vi "XCite_Only_Example.vi"() -> ()   [LabVIEW 2019]
doc: "This example demonstrates basic control of an X-Cite® light source. The first four channels of a connected light source can be switched on or off, and the power level adjusted. Note that this example will not be fail save, i.e. doesnt react on errors, just handles them forward to the end\n\nUsage:\n\nA search for X-Cite® devices is started, and if found controls are initialized for each channel. Channels can be switched on and off, and the intensity adjusted. To end the program click on \"quit\". All X-Cite® channels are switched off on exit."
uses:
  xcite/Xcite.lvclass
panel:
  out "error_out":errorcluster {"code" format="%.0x"}
  in  "quit":bool
  out "number_of_channels":i32
  in  "Power4":dbl
  out "Wavelength4":u32
  in  "Channel4":bool caption="wavelength"
  in  "Power3":dbl
  out "Wavelength3":u32
  in  "Channel3":bool caption="wavelength"
  in  "Power2":dbl
  out "Wavelength2":u32
  in  "Channel2":bool caption="wavelength"
  in  "Power1":dbl
  out "Wavelength1":u32
  in  "Channel1":bool caption="wavelength"
  out "display_name":string
  # "This example demonstrates basic control of an X-Cite® light source. The first four channels of a connected light source can be switched on or off, and the power level adjusted. Note that this example will not be fail save, i.e. doesnt react on errors, just handles them forward to the end\n\nUsage:\n\nA search for X-Cite® devices is started, and if found controls are initialized for each channel. Channels can be switched on and off, and the intensity adjusted. To end the program click on \"quit\". All X-Cite® channels are switched off on exit."
  # "pco.labview"
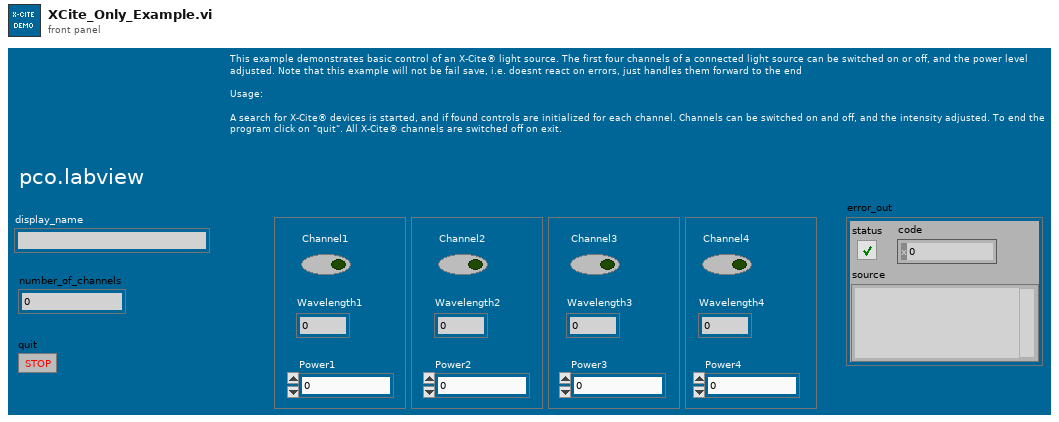
[diagram p1: front panel]
types:
  T1 = cluster{"serial":u32, "type":u16, "name":string, "wavelenghts_vec":u32[], "exclusivity_vec":u32[], "intensity_max_vec":u32[], "intensity_min_vec":u32[]}
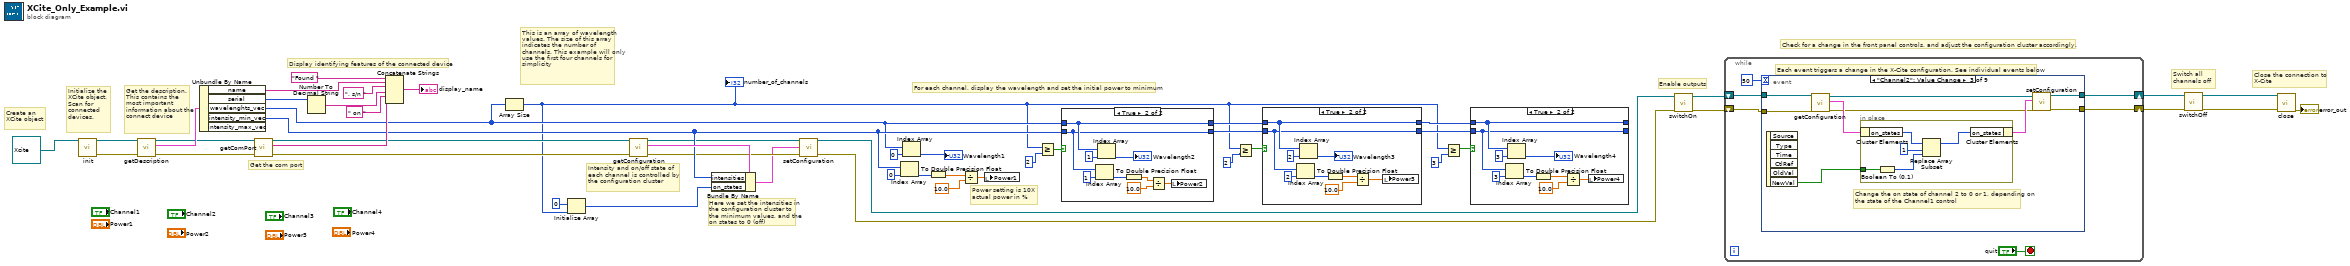
[diagram p0: block diagram]
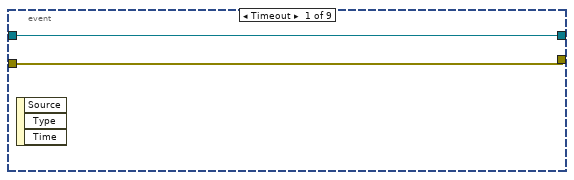
[diagram p2: hidden frame]
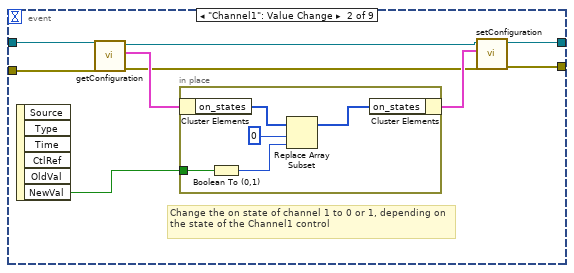
[diagram p3: hidden frame]
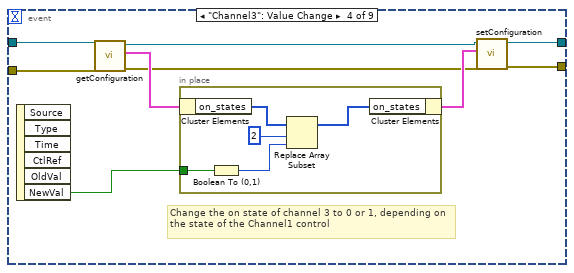
[diagram p4: hidden frame]
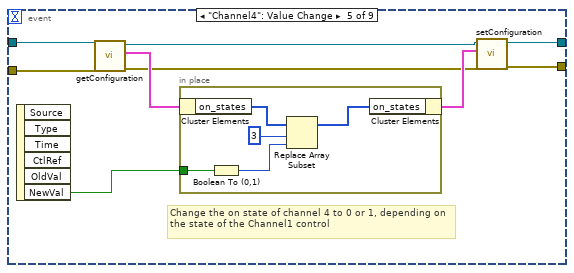
[diagram p5: hidden frame]
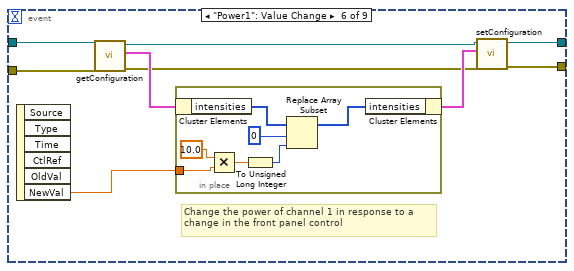
[diagram p6: hidden frame]
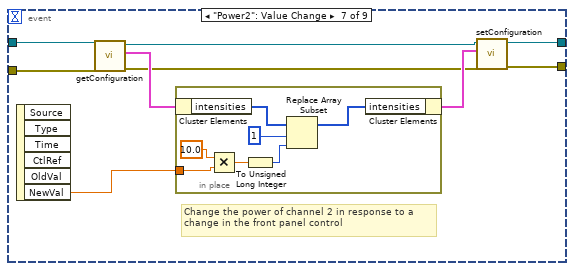
[diagram p7: hidden frame]
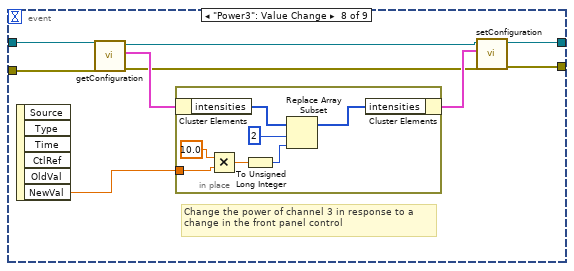
[diagram p8: hidden frame]
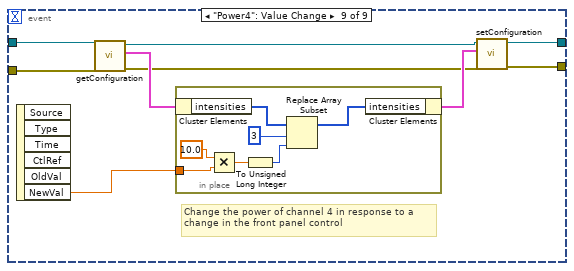
[diagram p9: hidden frame]
diagram:
  # "Enable outputs"
  # "Close the connection to X-Cite"
  # "Switch all channels off"
  # "Check for a change in the front panel controls, and adjust the configuration cluster accordingly."
  # "Power setting is 10X actual power in %"
  # "Here we set the intensities in the configuration cluster to the minimum values, and the on states to 0 (off)"
  # "Intensity and on/off state of each channel is controlled by the configuration cluster"
  # "For each channel, display the wavelength and set the initial power to minimum"
  # "This is an array of wavelength values. The size of this array indicates the number of channels. This example will only use the first four channels for simplicity"
  # "Display identifying features of the connected device"
  # "Get the com port"
  # "Get the description. This contains the most important information about the connect device"
  # "Initialize the XCite object. Scan for connected devices."
  # "Create an XCite object"
  n1 = call "init.vi"("Xcite in"=refnum<class "Xcite.lvclass"> refnum ("Xcite.lvclass")) -> ("error out"=w49:errorcluster, "Xcite out"=w50:refnum<class "Xcite.lvclass">)  [unwired: 9 in]
  n2 = call "getDescription.vi"("error in (no error)"=w49, "Xcite in"=w50) -> ("error out"=w45:errorcluster, "description"=w48:T1, "Xcite out"=w44:refnum<class "Xcite.lvclass">)  [unwired: 7 in]
  n3 = Unbundle By Name(w48) -> ("name"=w47:string, "serial"=w42:u32, "wavelenghts_vec"=w15:u32[], "intensity_min_vec"=w19:u32[])  [unwired: 1 out]
  n4 = call "getComPort.vi"("error in (no error)"=w45, "Xcite in"=w44) -> ("error out"=w21:errorcluster, "com_port"=w39:string, "Xcite out"=w22:refnum<class "Xcite.lvclass">)  [unwired: 7 in]
  n5 = Number To Decimal String(number=w42) -> (decimal integer string=w41:string)  [unwired: 1 in]
  n6 = Concatenate Strings("Found ", w47, ", s/n " ("string"), w41, " on " ("string"), w39) -> (→"display_name":string)
  n7 = Array Size(array=w15) -> (size(s)=w13:i32)
  "number_of_channels" <- w13
  n8 = Initialize Array(u8 0, w13) -> (w12:u8[])
  n9 = call "getConfiguration.vi"("error in (no error)"=w21, "Xcite in"=w22) -> ("error out"=w17:errorcluster, "configuration"=w20:cluster{"intensities":u32[], "on_states":u8[]}, "Xcite out"=w18:refnum<class "Xcite.lvclass">)  [unwired: 7 in]
  n10 = Bundle By Name(cluster=w20, "intensities"=w19, "on_states"=w12) -> (w16:cluster{"intensities":u32[], "on_states":u8[]})
  n11 = call "setConfiguration.vi"("error in (no error)"=w17, "configuration"=w16, "Xcite in"=w18) -> ("error out"=w2:errorcluster, "Xcite out"=w4:refnum<class "Xcite.lvclass">)  [unwired: 7 in]
  n12 = Index Array(array=w19, index=0) -> (element=w34:u32)
  n13 = Index Array(array=w15, index=0) -> (element=→"Wavelength1":u32)
  n14 = To Double Precision Float(number=w34) -> (double precision float=w33:dbl)
  n15 = Divide(x=w33, y=10.0) -> (x/y=w11:dbl)
  n16 = local write "Power1"(w11) -> ()
  n17 = Greater Or Equal?(x=w13, y=2) -> (x >= y?=w31:bool)
  n18 = case shown="True" w31 {
    tunnel: w15 -> [w53 w58]
    tunnel: w19 -> [w52 w57]
    tunnel: [w53 w58] -> w30
    tunnel: [w52 w57] -> w29
    frame False {
    }
    frame True {
      n19 = Index Array(array=w57, index=1) -> (element=w62:u32)
      n20 = Index Array(array=w58, index=1) -> (element=→"Wavelength2":u32)
      n21 = To Double Precision Float(number=w62) -> (double precision float=w55:dbl)
      n22 = Divide(x=w55, y=10.0) -> (x/y=w56:dbl)
      n23 = local write "Power2"(w56) -> ()
    }
  }
  n24 = Greater Or Equal?(x=w13, y=2) -> (x >= y?=w27:bool)
  n25 = case shown="True" w27 {
    tunnel: w30 -> [w64 w70]
    tunnel: w29 -> [w63 w69]
    tunnel: [w64 w70] -> w24
    tunnel: [w63 w69] -> w23
    frame False {
    }
    frame True {
      n26 = Index Array(array=w69, index=2) -> (element=w73:u32)
      n27 = Index Array(array=w70, index=2) -> (element=→"Wavelength3":u32)
      n28 = To Double Precision Float(number=w73) -> (double precision float=w68:dbl)
      n29 = Divide(x=w68, y=10.0) -> (x/y=w66:dbl)
      n30 = local write "Power3"(w66) -> ()
    }
  }
  n31 = Greater Or Equal?(x=w13, y=3) -> (x >= y?=w26:bool)
  n32 = case shown="True" w26 {
    tunnel: w24 -> [w75 w81]
    tunnel: w23 -> [w74 w80]
    tunnel: [w75 w81] -> _
    tunnel: [w74 w80] -> _
    frame False {
    }
    frame True {
      n33 = Index Array(array=w80, index=3) -> (element=w84:u32)
      n34 = Index Array(array=w81, index=3) -> (element=→"Wavelength4":u32)
      n35 = To Double Precision Float(number=w84) -> (double precision float=w77:dbl)
      n36 = Divide(x=w77, y=10.0) -> (x/y=w78:dbl)
      n37 = local write "Power4"(w78) -> ()
    }
  }
  n38 = call "switchOn.vi"("error in (no error)"=w2, "Xcite in"=w4) -> ("error out"=w1:errorcluster, "Xcite out"=w3:refnum<class "Xcite.lvclass">)  [unwired: 8 in]
  n39 = while {
    shift-right: [w86] -> w9
    shift-left: w3 -> [w87]
    shift-right: [w85] -> w8
    shift-left: w1 -> [w88]
    stop <- "quit" stop-if-true
    # "Each event triggers a change in the X-Cite configuration. See individual events below"
    n40 = event shown="[2] \"Channel2\": Value Change" {
      selector: _ -> [_ _ _ _ _ _ _ _ _]
      dyn-events: _ -> [_ _ _ _ _ _ _ _ _]
      timeout: 50 -> [_ _ _ _ _ _ _ _ _]
      tunnel: w88 -> [w91 w100 w114 w128 w142 w156 w172 w188 w204]
      tunnel: w87 -> [w92 w101 w115 w129 w143 w157 w173 w189 w205]
      tunnel: [w92 w94 w108 w122 w136 w150 w166 w182 w198] -> w86
      tunnel: [w91 w93 w107 w121 w135 w149 w165 w181 w197] -> w85
      event Timeout {
        n41 = event-data() -> ()  [unwired: 1 in, 3 out]
      }
      event "Channel1": Value Change {
        # "Change the on state of channel 1 to 0 or 1, depending on the state of the Channel1 control"
        n42 = event-data() -> ("NewVal"=w98:bool)  [unwired: 1 in, 5 out]
        n43 = call "getConfiguration.vi"("error in (no error)"=w100, "Xcite in"=w101) -> ("error out"=w95:errorcluster, "configuration"=w99:cluster{"intensities":u32[], "on_states":u8[]}, "Xcite out"=w96:refnum<class "Xcite.lvclass">)  [unwired: 7 in]
        n44 = in-place {
          in-place-border: w98 -> [w104]
          n45 = in-place-cluster #1(w99) -> ("on_states"=w106:u8[])
          n46 = Boolean To (0,1)(Boolean=w104) -> (0, 1=w103:i16)
          n47 = Replace Array Subset(array=w106, new element=w103, index=0) -> (w102:u8[])
          n48 = in-place-cluster #1("on_states"=w102) -> (w97:cluster{"intensities":u32[], "on_states":u8[]})
        }
        n49 = call "setConfiguration.vi"("error in (no error)"=w95, "configuration"=w97, "Xcite in"=w96) -> ("error out"=w93:errorcluster, "Xcite out"=w94:refnum<class "Xcite.lvclass">)  [unwired: 7 in]
      }
      event "Channel2": Value Change {
        # "Change the on state of channel 2 to 0 or 1, depending on the state of the Channel1 control"
        n50 = event-data() -> ("NewVal"=w112:bool)  [unwired: 1 in, 5 out]
        n51 = call "getConfiguration.vi"("error in (no error)"=w114, "Xcite in"=w115) -> ("error out"=w109:errorcluster, "configuration"=w113:cluster{"intensities":u32[], "on_states":u8[]}, "Xcite out"=w110:refnum<class "Xcite.lvclass">)  [unwired: 7 in]
        n52 = in-place {
          in-place-border: w112 -> [w118]
          n53 = in-place-cluster #2(w113) -> ("on_states"=w120:u8[])
          n54 = Boolean To (0,1)(Boolean=w118) -> (0, 1=w117:i16)
          n55 = Replace Array Subset(array=w120, new element=w117, index=1) -> (w116:u8[])
          n56 = in-place-cluster #2("on_states"=w116) -> (w111:cluster{"intensities":u32[], "on_states":u8[]})
        }
        n57 = call "setConfiguration.vi"("error in (no error)"=w109, "configuration"=w111, "Xcite in"=w110) -> ("error out"=w107:errorcluster, "Xcite out"=w108:refnum<class "Xcite.lvclass">)  [unwired: 7 in]
      }
      event "Channel3": Value Change {
        # "Change the on state of channel 3 to 0 or 1, depending on the state of the Channel1 control"
        n58 = event-data() -> ("NewVal"=w126:bool)  [unwired: 1 in, 5 out]
        n59 = call "getConfiguration.vi"("error in (no error)"=w128, "Xcite in"=w129) -> ("error out"=w123:errorcluster, "configuration"=w127:cluster{"intensities":u32[], "on_states":u8[]}, "Xcite out"=w124:refnum<class "Xcite.lvclass">)  [unwired: 7 in]
        n60 = in-place {
          in-place-border: w126 -> [w132]
          n61 = in-place-cluster #3(w127) -> ("on_states"=w134:u8[])
          n62 = Boolean To (0,1)(Boolean=w132) -> (0, 1=w131:i16)
          n63 = Replace Array Subset(array=w134, new element=w131, index=2) -> (w130:u8[])
          n64 = in-place-cluster #3("on_states"=w130) -> (w125:cluster{"intensities":u32[], "on_states":u8[]})
        }
        n65 = call "setConfiguration.vi"("error in (no error)"=w123, "configuration"=w125, "Xcite in"=w124) -> ("error out"=w121:errorcluster, "Xcite out"=w122:refnum<class "Xcite.lvclass">)  [unwired: 7 in]
      }
      event "Channel4": Value Change {
        # "Change the on state of channel 4 to 0 or 1, depending on the state of the Channel1 control"
        n66 = event-data() -> ("NewVal"=w140:bool)  [unwired: 1 in, 5 out]
        n67 = call "getConfiguration.vi"("error in (no error)"=w142, "Xcite in"=w143) -> ("error out"=w137:errorcluster, "configuration"=w141:cluster{"intensities":u32[], "on_states":u8[]}, "Xcite out"=w138:refnum<class "Xcite.lvclass">)  [unwired: 7 in]
        n68 = in-place {
          in-place-border: w140 -> [w146]
          n69 = in-place-cluster #4(w141) -> ("on_states"=w148:u8[])
          n70 = Boolean To (0,1)(Boolean=w146) -> (0, 1=w145:i16)
          n71 = Replace Array Subset(array=w148, new element=w145, index=3) -> (w144:u8[])
          n72 = in-place-cluster #4("on_states"=w144) -> (w139:cluster{"intensities":u32[], "on_states":u8[]})
        }
        n73 = call "setConfiguration.vi"("error in (no error)"=w137, "configuration"=w139, "Xcite in"=w138) -> ("error out"=w135:errorcluster, "Xcite out"=w136:refnum<class "Xcite.lvclass">)  [unwired: 7 in]
      }
      event "Power1": Value Change {
        # "Change the power of channel 1 in response to a change in the front panel control"
        n74 = event-data() -> ("NewVal"=w154:dbl)  [unwired: 1 in, 5 out]
        n75 = call "getConfiguration.vi"("error in (no error)"=w156, "Xcite in"=w157) -> ("error out"=w151:errorcluster, "configuration"=w155:cluster{"intensities":u32[], "on_states":u8[]}, "Xcite out"=w152:refnum<class "Xcite.lvclass">)  [unwired: 7 in]
        n76 = in-place {
          in-place-border: w154 -> [w160]
          n77 = in-place-cluster #5(w155) -> ("intensities"=w164:u32[])
          n78 = Multiply(x=10.0, y=w160) -> (x*y=w159:dbl)
          n79 = To Unsigned Long Integer(number=w159) -> (unsigned 32bit integer=w158:u32)
          n80 = Replace Array Subset(array=w164, new element=w158, index=0) -> (w162:u32[])
          n81 = in-place-cluster #5("intensities"=w162) -> (w153:cluster{"intensities":u32[], "on_states":u8[]})
        }
        n82 = call "setConfiguration.vi"("error in (no error)"=w151, "configuration"=w153, "Xcite in"=w152) -> ("error out"=w149:errorcluster, "Xcite out"=w150:refnum<class "Xcite.lvclass">)  [unwired: 7 in]
      }
      event "Power2": Value Change {
        # "Change the power of channel 2 in response to a change in the front panel control"
        n83 = event-data() -> ("NewVal"=w170:dbl)  [unwired: 1 in, 5 out]
        n84 = call "getConfiguration.vi"("error in (no error)"=w172, "Xcite in"=w173) -> ("error out"=w167:errorcluster, "configuration"=w171:cluster{"intensities":u32[], "on_states":u8[]}, "Xcite out"=w168:refnum<class "Xcite.lvclass">)  [unwired: 7 in]
        n85 = in-place {
          in-place-border: w170 -> [w176]
          n86 = in-place-cluster #6(w171) -> ("intensities"=w180:u32[])
          n87 = Multiply(x=10.0, y=w176) -> (x*y=w175:dbl)
          n88 = To Unsigned Long Integer(number=w175) -> (unsigned 32bit integer=w174:u32)
          n89 = Replace Array Subset(array=w180, new element=w174, index=1) -> (w178:u32[])
          n90 = in-place-cluster #6("intensities"=w178) -> (w169:cluster{"intensities":u32[], "on_states":u8[]})
        }
        n91 = call "setConfiguration.vi"("error in (no error)"=w167, "configuration"=w169, "Xcite in"=w168) -> ("error out"=w165:errorcluster, "Xcite out"=w166:refnum<class "Xcite.lvclass">)  [unwired: 7 in]
      }
      event "Power3": Value Change {
        # "Change the power of channel 3 in response to a change in the front panel control"
        n92 = event-data() -> ("NewVal"=w186:dbl)  [unwired: 1 in, 5 out]
        n93 = call "getConfiguration.vi"("error in (no error)"=w188, "Xcite in"=w189) -> ("error out"=w183:errorcluster, "configuration"=w187:cluster{"intensities":u32[], "on_states":u8[]}, "Xcite out"=w184:refnum<class "Xcite.lvclass">)  [unwired: 7 in]
        n94 = in-place {
          in-place-border: w186 -> [w192]
          n95 = in-place-cluster #7(w187) -> ("intensities"=w196:u32[])
          n96 = Multiply(x=10.0, y=w192) -> (x*y=w191:dbl)
          n97 = To Unsigned Long Integer(number=w191) -> (unsigned 32bit integer=w190:u32)
          n98 = Replace Array Subset(array=w196, new element=w190, index=2) -> (w194:u32[])
          n99 = in-place-cluster #7("intensities"=w194) -> (w185:cluster{"intensities":u32[], "on_states":u8[]})
        }
        n100 = call "setConfiguration.vi"("error in (no error)"=w183, "configuration"=w185, "Xcite in"=w184) -> ("error out"=w181:errorcluster, "Xcite out"=w182:refnum<class "Xcite.lvclass">)  [unwired: 7 in]
      }
      event "Power4": Value Change {
        # "Change the power of channel 4 in response to a change in the front panel control"
        n101 = event-data() -> ("NewVal"=w202:dbl)  [unwired: 1 in, 5 out]
        n102 = call "getConfiguration.vi"("error in (no error)"=w204, "Xcite in"=w205) -> ("error out"=w199:errorcluster, "configuration"=w203:cluster{"intensities":u32[], "on_states":u8[]}, "Xcite out"=w200:refnum<class "Xcite.lvclass">)  [unwired: 7 in]
        n103 = in-place {
          in-place-border: w202 -> [w208]
          n104 = in-place-cluster #8(w203) -> ("intensities"=w212:u32[])
          n105 = Multiply(x=10.0, y=w208) -> (x*y=w207:dbl)
          n106 = To Unsigned Long Integer(number=w207) -> (unsigned 32bit integer=w206:u32)
          n107 = Replace Array Subset(array=w212, new element=w206, index=3) -> (w210:u32[])
          n108 = in-place-cluster #8("intensities"=w210) -> (w201:cluster{"intensities":u32[], "on_states":u8[]})
        }
        n109 = call "setConfiguration.vi"("error in (no error)"=w199, "configuration"=w201, "Xcite in"=w200) -> ("error out"=w197:errorcluster, "Xcite out"=w198:refnum<class "Xcite.lvclass">)  [unwired: 7 in]
      }
    }
  }
  n110 = call "switchOff.vi"("error in (no error)"=w8, "Xcite in"=w9) -> ("error out"=w6:errorcluster, "Xcite out"=w7:refnum<class "Xcite.lvclass">)  [unwired: 8 in]
  n111 = call "close.vi"("error in (no error)"=w6, "Xcite in"=w7) -> ("error out"=→"error_out":errorcluster)  [unwired: 9 in]
